vi "Hex to Ascii.vi"(11 "result string":string) -> (2 "Array":string[](array[string]), 3 "String":string)   [LabVIEW 2011, in "VIN.lvclass"]
uses:
  VIN.lvclass
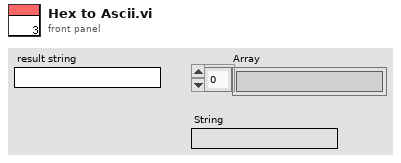
[diagram p1: front panel]
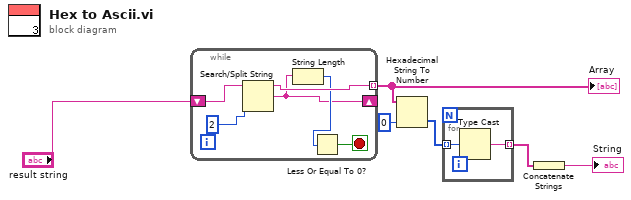
[diagram p0: block diagram]
diagram:
  n1 = while {
    shift-right: [w7] -> _
    shift-left: "result string" -> [w12]
    tunnel: [w11] -> w5 mode=indexing
    stop <- w9 stop-if-true
    n2 = Search/Split String(string=w12, offset (0)=2 ("y")) -> (substring before match=w11:string, match + rest of string=w7:string)  [unwired: 1 in, 1 out]
    n3 = String Length(string=w7) -> (length=w10:i32)
    n4 = Less Or Equal To 0?(x=w10) -> (x <= 0?=w9:bool)
  }
  "Array" <- w5
  n5 = Hexadecimal String To Number(string=w5, default (0uL)=u8 0 ("default (0 U32)")) -> (number=w6:u8[])  [unwired: 1 in, 1 out]
  n6 = for {
    tunnel: [w14] -> w3 mode=indexing
    tunnel: w6 -> [w13] mode=indexing
    n7 = Type Cast(x=w13) -> (*(type *) &x=w14:string)  [unwired: 1 in]
  }
  n8 = Concatenate Strings(w3) -> (→"String":string)
